vi "Distance Between Points.vi"(4 "B":cluster{"x":dbl, "y":dbl}, 5 "A":cluster{"x":dbl, "y":dbl}) -> (1 "distance":dbl)   [LabVIEW 2020]
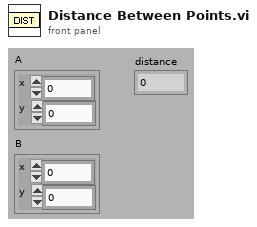
[diagram p1: front panel]
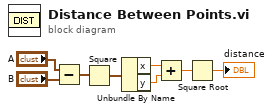
[diagram p0: block diagram]
diagram:
  n1 = Subtract(x="A", y="B") -> (x-y=w6:cluster{"x":dbl, "y":dbl})
  n2 = Square(x=w6) -> (x^2=w5:cluster{"x":dbl, "y":dbl})
  n3 = Unbundle By Name(w5) -> ("x"=w4:dbl, "y"=w3:dbl)
  n4 = Add(x=w4, y=w3) -> (x+y=w2:dbl)
  n5 = Square Root(x=w2) -> (sqrt(x)=→"distance":dbl)
